vi "DIAdem Application Start.vi"(4 "DIAdem Additional Start Parameters":string, 5 "DIAdem Command":string, 6 "error in (no error)":errorcluster, 7 "DIAdem Desktop File":path, 8 "DIAdem System Directory":path, 9 "DIAdem Directory":path) -> (0 "error out":errorcluster)   [LabVIEW 2020]
doc: "This VI starts DIAdem."
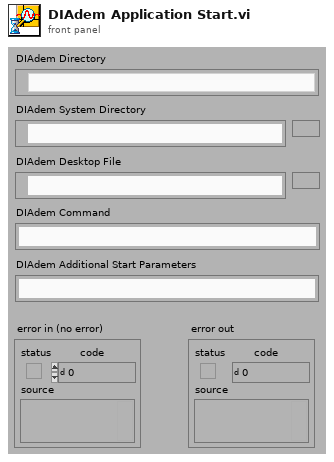
[diagram p1: front panel]
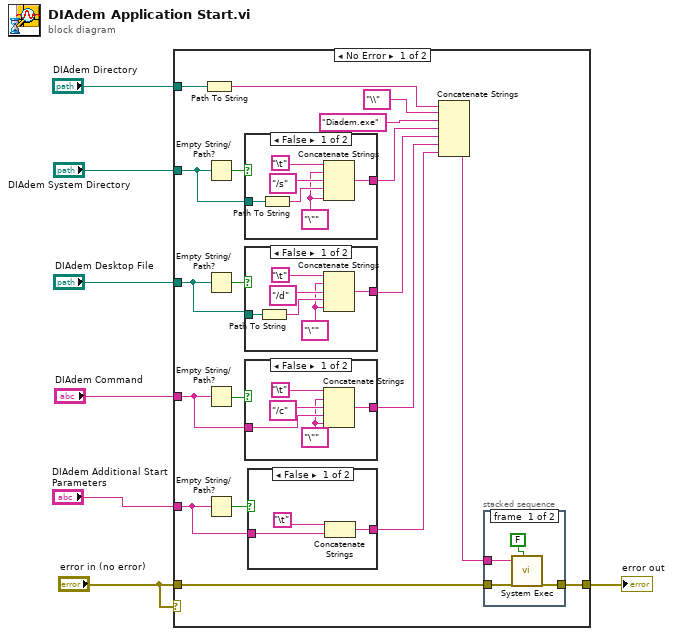
[diagram p0: block diagram]
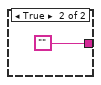
[diagram p2: hidden frame]
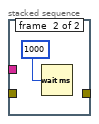
[diagram p3: hidden frame]
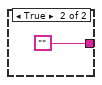
[diagram p4: hidden frame]
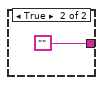
[diagram p5: hidden frame]
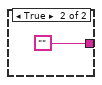
[diagram p6: hidden frame]
diagram:
  n1 = case shown="No Error" "error in (no error)" {
    tunnel: "DIAdem Desktop File" -> [w19 _]
    tunnel: "DIAdem Directory" -> [w20 _]
    tunnel: "DIAdem Command" -> [w18 _]
    tunnel: [w14 w56] -> w4
    tunnel: "error in (no error)" -> [w13 w56]
    tunnel: "DIAdem Additional Start Parameters" -> [w15 _]
    tunnel: "DIAdem System Directory" -> [w11 _]
    frame No Error {
      n2 = Path To String(path=w20) -> (string=w25:string)
      n3 = Empty String/Path?(string/path=w11) -> (empty?=w12:bool)
      n4 = Empty String/Path?(string/path=w19) -> (empty?=w26:bool)
      n5 = Empty String/Path?(string/path=w18) -> (empty?=w22:bool)
      n6 = Empty String/Path?(string/path=w15) -> (empty?=w17:bool)
      n7 = case shown="False" w12 {
        tunnel: [w32 ""] -> w9
        tunnel: w11 -> [w31 _]
        frame False {
          w27 = "\"" ("Substring")
          n8 = Path To String(path=w31) -> (string=w30:string)
          n9 = Concatenate Strings("\t", w27, "/s" ("Substring"), w30, w27) -> (w32:string)
        }
        frame True {
        }
      }
      n10 = case shown="False" w26 {
        tunnel: [w53 ""] -> w10
        tunnel: w19 -> [w52 _]
        frame False {
          w49 = "\"" ("Substring")
          n11 = Path To String(path=w52) -> (string=w54:string)
          n12 = Concatenate Strings("\t", w49, "/d" ("Substring"), w54, w49) -> (w53:string)
        }
        frame True {
        }
      }
      n13 = case shown="False" w22 {
        tunnel: [w47 ""] -> w21
        tunnel: w18 -> [w45 _]
        frame False {
          w43 = "\"" ("Substring")
          n14 = Concatenate Strings("\t", w43, "/c" ("Substring"), w45, w43) -> (w47:string)
        }
        frame True {
        }
      }
      n15 = case shown="False" w17 {
        tunnel: [w41 ""] -> w16
        tunnel: w15 -> [w39 _]
        frame False {
          n16 = Concatenate Strings("\t", w39) -> (w41:string)
        }
        frame True {
        }
      }
      n17 = Concatenate Strings(w25, "\\" ("Substring"), "Diadem.exe", w9, w10, w21, w16) -> (w8:string)
      n18 = stacked-sequence {
        tunnel: w13 -> [w36 _]
        tunnel: w8 -> [w35 _]
        tunnel: [w34 _] -> w14
        frame #0 {
          n19 = call <vilib>:"System Exec.vi"("wait until completion? (T)"=FALSE, "error in (no error)"=w36, "command line"=w35) -> ("error out"=w34:errorcluster)  [unwired: 5 in, 3 out]
        }
        frame #1 {
          n20 = Wait (ms)(milliseconds to wait=u32 1000) -> ()  [unwired: 1 out]
        }
      }
    }
    frame Error {
    }
  }
  "error out" <- w4
